vi "Exercise 3-5.vi"() -> ()   [LabVIEW 2014]
panel:
  out "Warning?":bool
  out "Warning Text":string
  in  "Min Temp":dbl
  in  "Max Temp":dbl
  in  "Current Temp":dbl
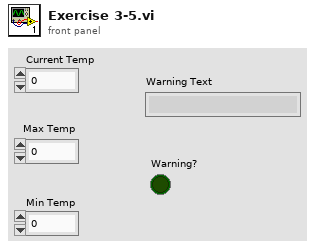
[diagram p1: front panel]
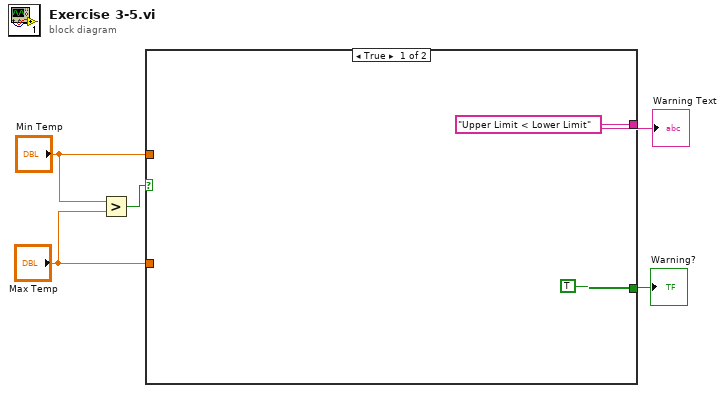
[diagram p0: block diagram]
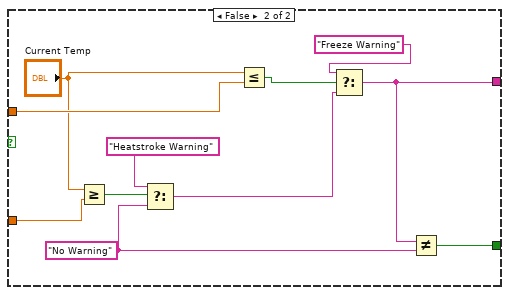
[diagram p2: hidden frame]
diagram:
  n1 = Greater?(x="Min Temp", y="Max Temp") -> (0:w3:bool)
  n2 = case shown="True" w3 {
    tunnel: [TRUE w16] -> w5
    tunnel: ["Upper Limit < Lower Limit" w15] -> w4
    tunnel: "Max Temp" -> [_ w13]
    tunnel: "Min Temp" -> [_ w11]
    frame True {
    }
    frame False {
      w8 = "No Warning" ("String")
      n3 = Greater Or Equal?(x="Current Temp", y=w13) -> (x >= y?=w9:bool)
      n4 = Select(t="Heatstroke Warning" ("String"), s=w9, f=w8) -> (s? t:f=w14:string)
      n5 = Less Or Equal?(x="Current Temp", y=w11) -> (x <= y?=w18:bool)
      n6 = Select(t="Freeze Warning" ("String"), s=w18, f=w14) -> (s? t:f=w15:string)
      n7 = Not Equal?(x=w15, y=w8) -> (x != y?=w16:bool)
    }
  }
  "Warning Text" <- w4
  "Warning?" <- w5
